vi "Test 6.vi"(8 "error in (no error)":errorcluster, 11 "Test Case In":refnum<class "Tests.lvclass">) -> (0 "error out":errorcluster, 3 "Test Case Out":refnum<class "Tests.lvclass">)   [LabVIEW 2021, in "Tests.lvclass"]
uses:
  Tests.lvclass
  C:/Program Files (x86)/National Instruments/LabVIEW 2021/vi.lib/Astemes/LUnit/Test Case.lvclass
  <vilib>/Astemes/LUnit/Test Case.lvclass/Test Case.ctl
  <vilib>/Astemes/LUnit/Append Fail Result.vi
  <vilib>/Astemes/LUnit/Append Pass Result.vi
  Proto/Hailstone.lvclass
  <vilib>/Astemes/LUnit/Test Case.lvclass
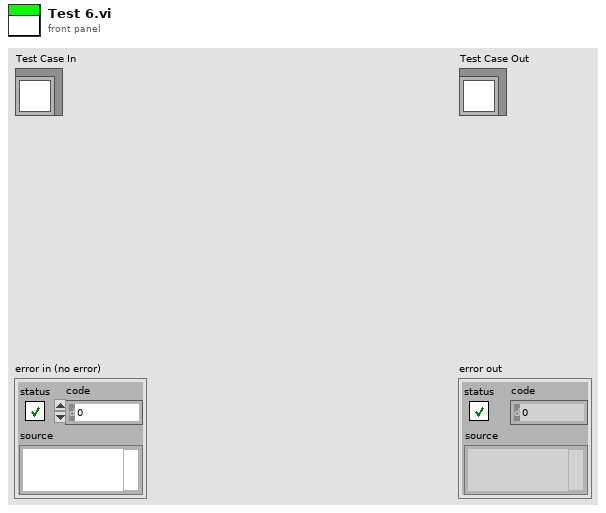
[diagram p1: front panel]
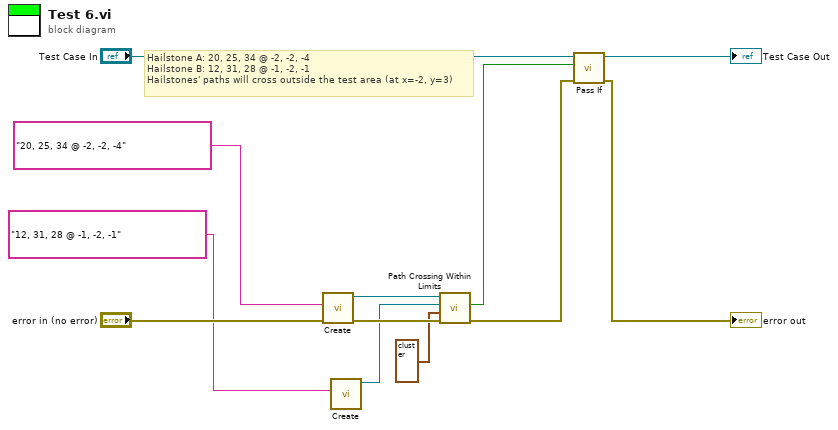
[diagram p0: block diagram]
diagram:
  # "Hailstone A: 20, 25, 34 @ -2, -2, -4\nHailstone B: 12, 31, 28 @ -1, -2, -1\nHailstones' paths will cross outside the test area (at x=-2, y=3)"
  n1 = call "Create.vi"("error in (no error)"="error in (no error)", "Input"="20, 25, 34 @ -2, -2, -4") -> ("error out"=w8:errorcluster, "Hailstone Out"=w6:refnum<class "Hailstone.lvclass">)  [unwired: 8 in]
  n2 = call "Create.vi"("Input"="12, 31, 28 @ -1, -2, -1") -> ("Hailstone Out"=w3:refnum<class "Hailstone.lvclass">)  [unwired: 9 in, 1 out]
  n3 = call "Path Crossing Within Limits.vi"("error in (no error)"=w8, "Limits"=cluster{"Min":ext, "Max":ext} {"Min"=-2.0, "Max"=3.0}, "Hailstone 2"=w3, "Hailstone In"=w6) -> ("error out"=w7:errorcluster, "Crossing?"=w1:bool)  [unwired: 5 in, 1 out]
  n4 = call <vilib>:"Pass If.vi"("error in (no error)"=w7, "Pass?"=w1, "LUnit Test Case In"="Test Case In") -> ("error out"=→"error out":errorcluster, "LUnit Test Case Out"=→"Test Case Out":refnum<class "Tests.lvclass">)  [unwired: 7 in]
